vi "uintDivide.vi"(8 "Error in (no error)":errorcluster, 10 "Uint2 in":refnum<class "UintClass.lvclass">, 11 "Uint1 in":refnum<class "UintClass.lvclass">) -> (0 "Error out":errorcluster, 1 "Timing":u32, 2 "floor(Uint1/Uint2)":refnum<class "UintClass.lvclass">, 3 "Uint1 mod Uint2":refnum<class "UintClass.lvclass">)   [LabVIEW 2011, in "UintClass.lvclass"]
uses:
  UintClass.lvclass
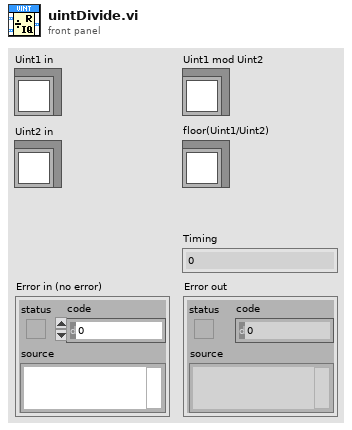
[diagram p1: front panel]
types:
  T1 = typedef "UintClass.lvclass/enumBase.ctl" = u16
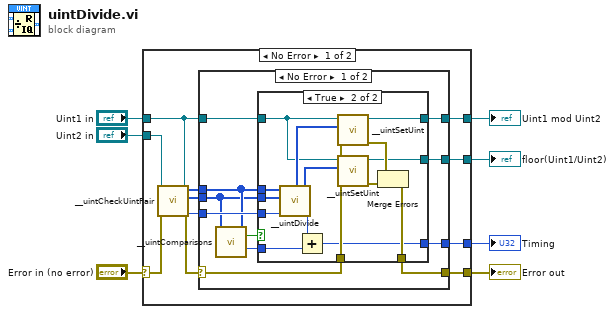
[diagram p0: block diagram]
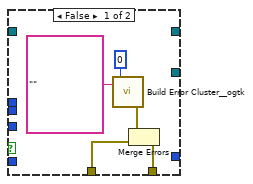
[diagram p2: hidden frame]
diagram:
  n1 = case shown="No Error" "Error in (no error)" {
    selector: "Error in (no error)" -> [w15 w51]
    tunnel: [w13 w51] -> w6
    tunnel: "Uint2 in" -> [w16 _]
    tunnel: "Uint1 in" -> [w9 _]
    tunnel: [w18 _] -> w3
    tunnel: [w17 _] -> w2
    tunnel: [w8 _] -> w1
    frame No Error {
      n2 = call "__uintCheckUintPair.vi"("Error in (no error)"=w15, "Uint2 in"=w16, "Uint1 in"=w9) -> ("Error out"=w14:errorcluster, "Uint2 out"=w11:u8[], "Uint1 out"=w12:u8[], "Base out"=w10:T1)  [unwired: 5 in]
      n3 = case shown="No Error" w14 {
        selector: w14 -> [w25 w50]
        tunnel: [w29 _] -> w18
        tunnel: [w28 _] -> w17
        tunnel: [w24 w50] -> w13
        tunnel: w12 -> [w23 _]
        tunnel: w11 -> [w22 _]
        tunnel: w10 -> [w27 _]
        tunnel: w9 -> [w26 _]
        tunnel: [w21 _] -> w8
        frame No Error {
          n4 = call "__uintComparisons.vi"("Uint2 in"=w22, "Uint1 in"=w23) -> ("Timing comparison"=w19:u32, "Uint1 > Uint2"=w20:bool)  [unwired: 3 in, 5 out]
          n5 = case shown="True" w20 {
            tunnel: [_ w37] -> w29
            tunnel: [_ w48] -> w28
            tunnel: w27 -> [_ w47]
            tunnel: w26 -> [_ w40]
            tunnel: w25 -> [w34 w44]
            tunnel: [w33 w41] -> w24
            tunnel: w23 -> [_ w46]
            tunnel: w22 -> [_ w45]
            tunnel: [_ w38] -> w21
            tunnel: w19 -> [_ w35]
            frame False {
              n6 = call <userlib>:"Build Error Cluster__ogtk.vi"("String to Prepend to source (\"\")"="" ("String to Prepend to source (\"\")"), "code"=0) -> ("error out"=w32:errorcluster)
              n7 = Merge Errors(w32, w34) -> (w33:errorcluster)
            }
            frame True {
              n8 = call "__uintDivide.vi"("Base (decimal)"=w47, "Uint2 in"=w45, "Uint1 in"=w46) -> ("Timing division"=w36:u32, "floor(Uint1 / Uint1)"=w39:u8[], "Uint1 mod Uint2"=w49:u8[])  [unwired: 6 in]
              n9 = Add(x=w36, y=w35) -> (x+y=w37:u32)
              n10 = call "__uintSetUint.vi"("Error in (no error)"=w44, 10:"Uint in"=w49, 11:"Uint in"=w40) -> ("Error out"=w43:errorcluster, "Uint out"=w48:refnum<class "UintClass.lvclass">)  [unwired: 7 in]
              n11 = call "__uintSetUint.vi"("Error in (no error)"=w44, 10:"Uint in"=w39, 11:"Uint in"=w40) -> ("Error out"=w42:errorcluster, "Uint out"=w38:refnum<class "UintClass.lvclass">)  [unwired: 7 in]
              n12 = Merge Errors(w43, w42) -> (w41:errorcluster)
            }
          }
        }
        frame Error {
        }
      }
    }
    frame Error {
    }
  }
  "Error out" <- w6
  "Uint1 mod Uint2" <- w2
  "Timing" <- w3
  "floor(Uint1/Uint2)" <- w1
